vi "NT Local Server.vi"   [LabVIEW 2013]
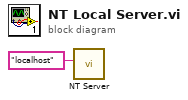
[diagram p0: block diagram]
diagram:
  n1 = call <vilib>:"NT Server.vi"("Server Name"="localhost") -> ()  [unwired: 11 in]
